vi "dvp Vi Get Bayer Decode Sel Detail.vi"(7 "pIndex":i32, 9 "pBayerDecodeSelDetailString":string, 10 "BayerDecodeSel":u32, 11 "handle":u32) -> (1 "pBayerDecodeSelDetailString out":string, 3 "function return":u32(ring), 5 "pIndex out":i32)   [LabVIEW 2018, in "LabViewDVPCamera.lvlib"]
doc: "LabviewDvp2Api dvpStatus dvpViGetBayerDecodeSelDetail(dvpHandle handle, dvpUint32 BayerDecodeSel, char* pBayerDecodeSelDetailString, dvpInt32 *pIndex);"
uses:
  LabViewDVPCamera.lvlib
  LabViewDVPCamera/LabViewDVPCamera.dll
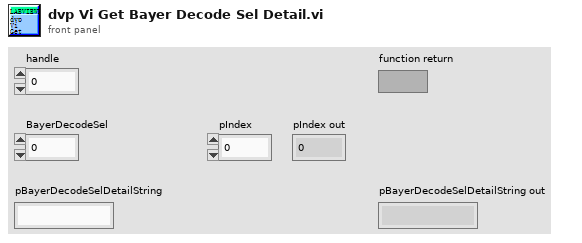
[diagram p1: front panel]
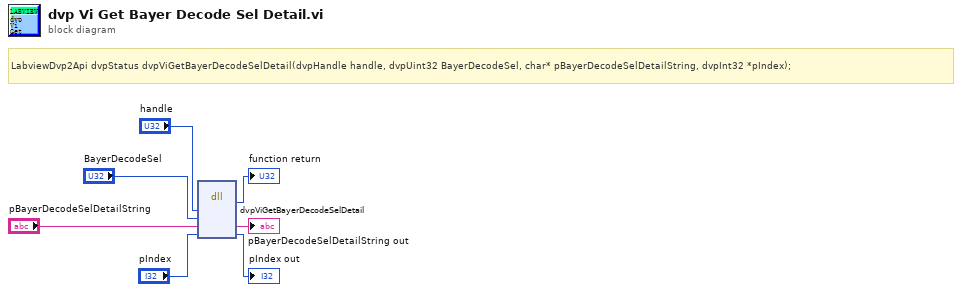
[diagram p0: block diagram]
diagram:
  # "LabviewDvp2Api dvpStatus dvpViGetBayerDecodeSelDetail(dvpHandle handle, dvpUint32 BayerDecodeSel, char* pBayerDecodeSelDetailString, dvpInt32 *pIndex);"
  n1 = dll-call lib="C:/Program Files (x86)/DVP2 Labview cn 64/Sample/LabViewDVPCamera/LabViewDVPCamera.*" fn="dvpViGetBayerDecodeSelDetail"("handle"="handle", "BayerDecodeSel"="BayerDecodeSel", "pBayerDecodeSelDetailString"="pBayerDecodeSelDetailString", "pIndex"="pIndex") -> (→"function return":u32, "pBayerDecodeSelDetailString"=→"pBayerDecodeSelDetailString out":string, "pIndex"=→"pIndex out":i32)  [unwired: 5 in, 2 out]
